vi "receiveDecodeAndDoKalman.vi"(0 "Vision in":refnum<class "Vision.lvclass">, 1 "cameras array":dbl[](array[numeric]), 3 "Ignore left/rigth?":bool[](array[boolean]), 5 "unsigned byte array":u8[](array[numeric]), 7 "Com UDP":T1={"UDP GrSim TX"=FALSE, "Address:"="127.0.0.1", "Port:"=20011}, 9 "Estimador":T7=enum."Nenhum", 10 "max ball vel":dbl, 11 "error in (no error)":errorcluster, 12 "team/side":u16[](array[numeric]), 13 "FIRASim?":bool=TRUE, 14 "Fps":dbl=40.0) -> (4 "Vision out":refnum<class "Vision.lvclass">, 6 "Frame and Field Size out":T2 {"Detection Frame Out"."robots_blue"."height" format="%+4.3f"; "Detection Frame Out"."robots_blue"."pixel_y" format="%+4.3f"; "Detection Frame Out"."robots_blue"."pixel_x" format="%+4.3f"; "Detection Frame Out"."robots_blue"."orientation" format="%+4.3f"; "Detection Frame Out"."robots_blue"."y" format="%+4.3f"; "Detection Frame Out"."robots_blue"."confidence" format="%4.3f"; "Detection Frame Out"."robots_blue"."x" format="%+4.3f"; "Detection Frame Out"."robots_yellow"."height" format="%+4.3f"; "Detection Frame Out"."robots_yellow"."pixel_y" format="%+4.3f"; "Detection Frame Out"."robots_yellow"."pixel_x" format="%+4.3f"; "Detection Frame Out"."robots_yellow"."orientation" format="%+4.3f"; "Detection Frame Out"."robots_yellow"."y" format="%+4.3f"; "Detection Frame Out"."robots_yellow"."confidence" format="%4.3f"; "Detection Frame Out"."robots_yellow"."x" format="%+4.3f"}, 15 "error out":errorcluster)   [LabVIEW 2023, in "Vision.lvclass"]
uses:
  Vision.lvclass
  Old vision/Controls/Estimadores.ctl
  Old vision/Controls/SSL Field State.ctl
  Old vision/Controls/SSL Detection Frame.ctl
  Old vision/Controls/SSL Detection Robot.ctl
  <vilib>/Analysis/Matrix/Datatypes/RealMatrix.ctl
  Old vision/Controls/SSL Detection Ball.ctl
  Controls/ComUDP.ctl
  <vilib>/Analysis/Matrix/NI_Matrix.lvlib
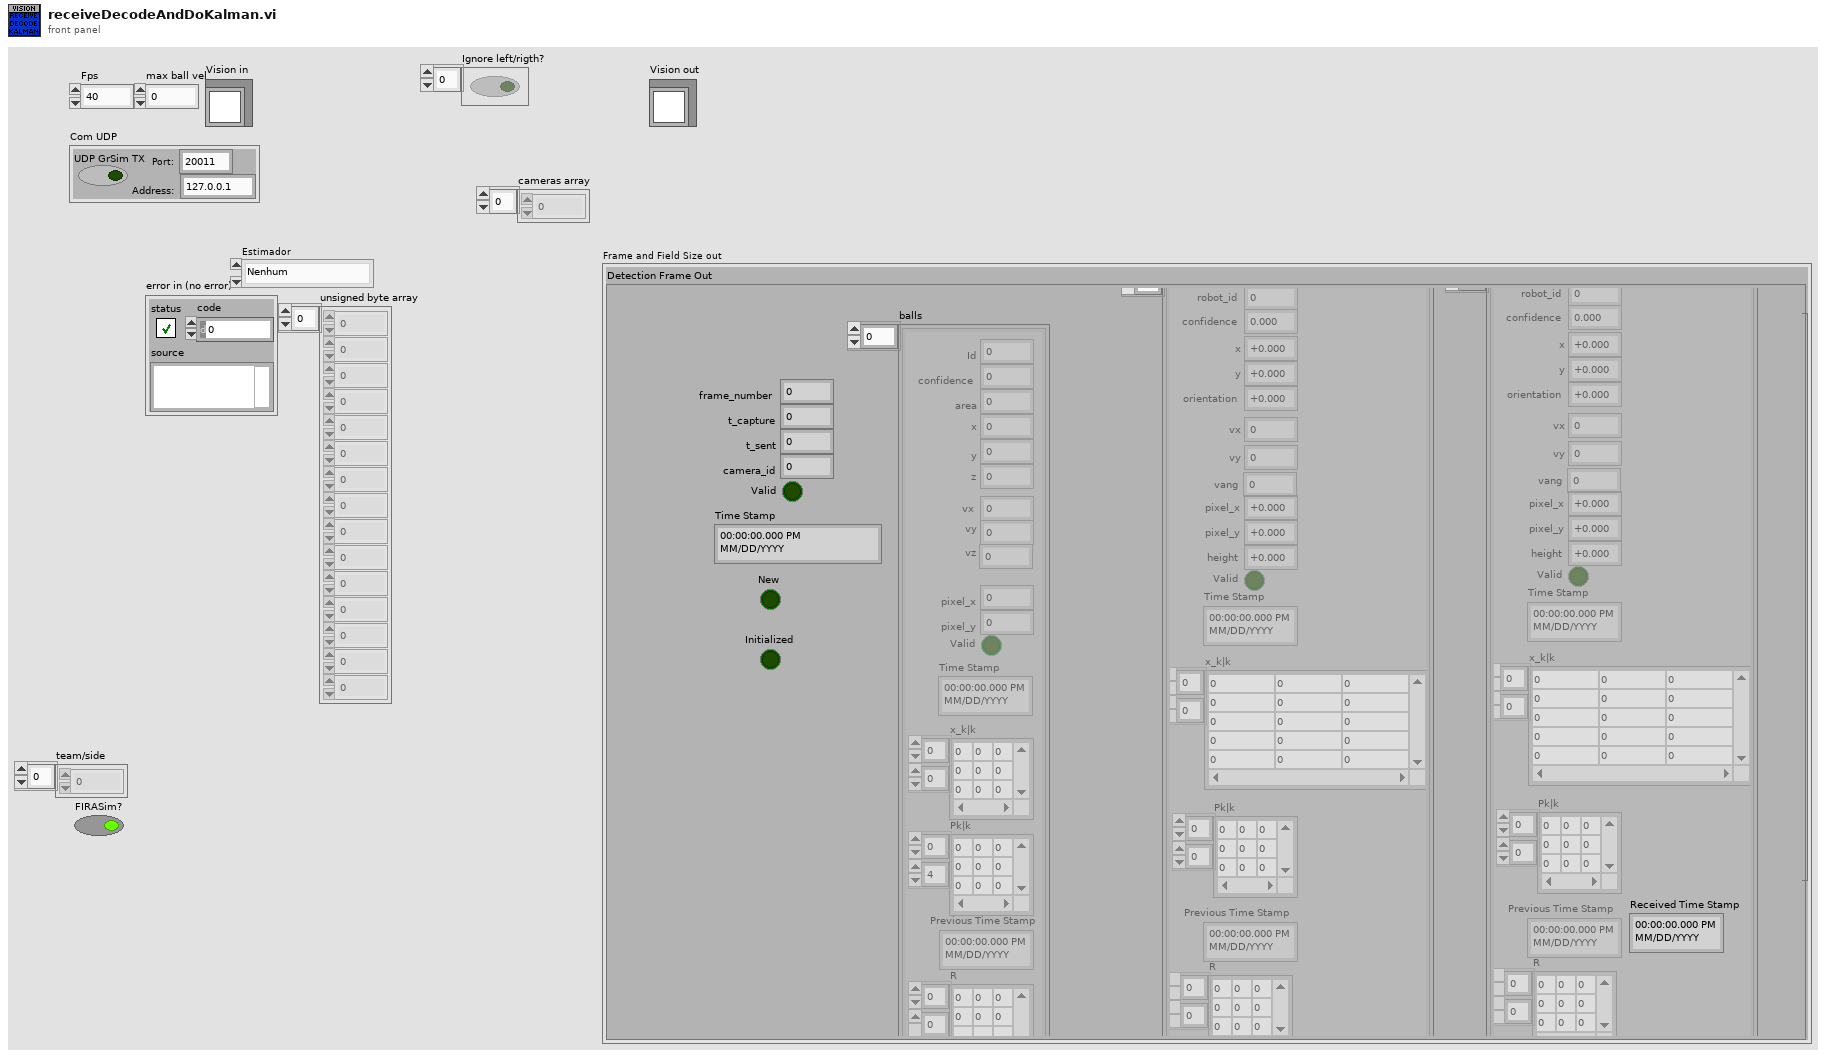
[diagram p1: front panel]
types:
  T1 = typedef "ComUDP.ctl" = cluster{"UDP GrSim TX":bool, "Address:":string, "Port:":u16}
  T2 = typedef "SSL Field State.ctl" = cluster{"Detection Frame Out":T3, "Field Size Out":cluster{"line_width":u32, "field_length":u32, "field_width":u32, "boundary_width":u32, "referee_width":u32, "goal_width":u32, "goal_depth":u32, "goal_wall_width":u32, "center_circle_radius":u32, "defense_radius":u32, "defense_stretch":u32, "free_kick_from_defense_dist":u32, "penalty_spot_from_field_line_dist":u32, "penalty_line_from_spot_dist":u32}, "Received Time Stamp":timestamp}
  T3 = typedef "SSL Detection Frame.ctl" = cluster{"frame_number":u32, "t_capture":dbl, "t_sent":dbl, "camera_id":u32, "robots_yellow":T4[], "robots_blue":T4[], "balls":T6[], "Valid":bool, "Time Stamp":timestamp, "New":bool, "Initialized":bool}
  T4 = typedef "SSL Detection Robot.ctl" = cluster{"x":sgl, "robot_id":u32, "confidence":sgl, "y":sgl, "orientation":sgl, "pixel_x":sgl, "pixel_y":sgl, "height":sgl, "Valid":bool, "Time Stamp":timestamp, "x_k|k":T5, "Pk|k":T5, "Previous Time Stamp":timestamp, "R":T5, "vx":dbl, "vy":dbl, "vang":dbl}
  T5 = typedef "NI_Matrix.lvlib/RealMatrix.ctl" = dbl[][]
  T6 = typedef "SSL Detection Ball.ctl" = cluster{"x":sgl, "area":u32, "confidence":sgl, "y":sgl, "z":sgl, "pixel_x":sgl, "pixel_y":sgl, "Valid":bool, "Time Stamp":timestamp, "x_k|k":T5, "Pk|k":T5, "Id":u32, "Previous Time Stamp":timestamp, "R":T5, " vx":sgl, "vy":dbl, "vz":dbl}
  T7 = typedef "Estimadores.ctl" = enum16{"4thDerivate", "2ndDerivate", "Nenhum", "Simples", "Kalman"}
  T8 = cluster{"line_width":u32, "field_length":u32, "field_width":u32, "boundary_width":u32, "referee_width":u32, "goal_width":u32, "goal_depth":u32, "goal_wall_width":u32, "center_circle_radius":u32, "defense_radius":u32, "defense_stretch":u32, "free_kick_from_defense_dist":u32, "penalty_spot_from_field_line_dist":u32, "penalty_line_from_spot_dist":u32}
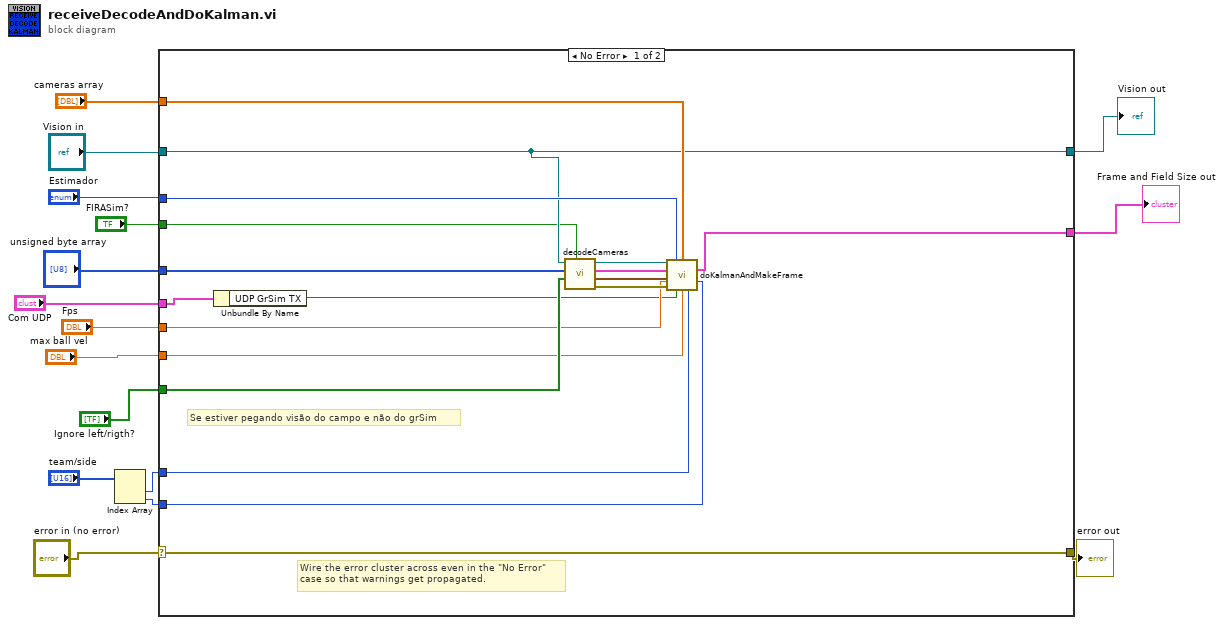
[diagram p0: block diagram]
diagram:
  n1 = Index Array(array="team/side") -> (element #1=w10:u16, element #2=w9:u16)  [unwired: 2 in]
  n2 = case shown="No Error" "error in (no error)" {
    selector: "error in (no error)" -> [w34 w36]
    tunnel: [w34 w36] -> w15
    tunnel: [w24 w35] -> w13
    tunnel: "Vision in" -> [w24 w35]
    tunnel: [w30 _] -> w12
    tunnel: w10 -> [w29 _]
    tunnel: w9 -> [w28 _]
    tunnel: "Estimador" -> [w27 _]
    tunnel: "cameras array" -> [w26 _]
    tunnel: "Ignore left/rigth?" -> [w25 _]
    tunnel: "unsigned byte array" -> [w23 _]
    tunnel: "Fps" -> [w22 _]
    tunnel: "Com UDP" -> [w21 _]
    tunnel: "max ball vel" -> [w18 _]
    tunnel: "FIRASim?" -> [w17 _]
    frame No Error {
      # "Se estiver pegando visão do campo e não do grSim"
      # "Wire the error cluster across even in the \"No Error\"\ncase so that warnings get propagated."
      n3 = Unbundle By Name(w21) -> ("UDP GrSim TX"=w20:bool)
      n4 = call "decodeCameras.vi"("FIRASim?"=w17, "Ignore left/rigth?"=w25, "unsigned byte array"=w23, "Vision in"=w24) -> ("error out"=w31:errorcluster, "Field Size"=w32:T8, "Detection Frame"=w19:T3, "Vision out"=w33:refnum<class "Vision.lvclass">)  [unwired: 1 in, 3 out]
      n5 = call "doKalmanAndMakeFrame.vi"("Vision in"=w33, "Estimador"=w27, "cameras array"=w26, "Detection Frame"=w19, "Field Size"=w32, "Fps"=w22, "Side"=w28, "error in (no error)"=w31, "grSim"=w20, "max ball vel"=w18, "Team"=w29) -> ("Frame and Field Size out"=w30:T2)  [unwired: 2 in, 2 out]
    }
    frame Error {
    }
  }
  "error out" <- w15
  "Vision out" <- w13
  "Frame and Field Size out" <- w12
